vi "Normalize 1D float array.vi"(10 "Signal treat":T1(ring), 11 "Data in":sgl[](array[numeric])) -> (3 "Data out":sgl[](array[numeric]))   [LabVIEW 2021, in "MatS Libs.lvlib"]
doc: "Scales signal in 1D array of single precision numbers.\nFor double precision, you can use Scale.vi, Quick scale.vi or Normalize.vi from Signal processing palete."
uses:
  <userlib>/_MGI/1D Array/MGI Average/MGI Average (SGL[]).vi
  <userlib>/MatS Libs/MatS Libs.lvlib
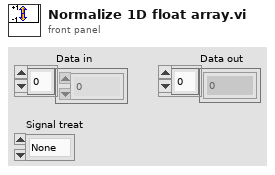
[diagram p1: front panel]
types:
  T1 = enum16{"None", "Unity norm", "Mean norm", "Standardization"}
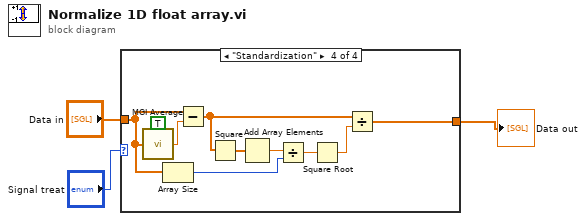
[diagram p0: block diagram]
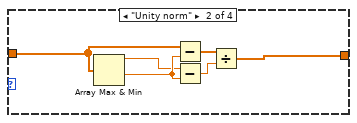
[diagram p3: hidden frame]
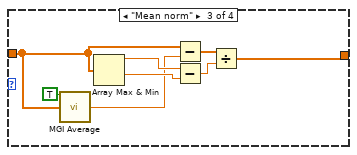
[diagram p4: hidden frame]
diagram:
  n1 = case shown="\"Standardization\"" "Signal treat" {
    tunnel: [w4 w8 w13 w26] -> w3
    tunnel: "Data in" -> [w4 w10 w16 w23]
    frame "None", Default {
      # "No feature scaling"
    }
    frame "Unity norm" {
      n2 = Array Max & Min(array=w10) -> (max value=w7:sgl, min value=w9:sgl)  [unwired: 2 out]
      n3 = Subtract(x=w10, y=w9) -> (x-y=w6:sgl[])
      n4 = Subtract(x=w7, y=w9) -> (x-y=w5:sgl)
      n5 = Divide(x=w6, y=w5) -> (x/y=w8:sgl[])
    }
    frame "Mean norm" {
      n6 = call-poly <userlib>:"MGI Average.vi"("Single[]"=w16, "Ignore NaN? (F)"=TRUE) -> ("Average"=w15:sgl)
      n7 = Array Max & Min(array=w16) -> (max value=w17:sgl, min value=w18:sgl)  [unwired: 2 out]
      n8 = Subtract(x=w16, y=w15) -> (x-y=w12:sgl[])
      n9 = Subtract(x=w17, y=w18) -> (x-y=w11:sgl)
      n10 = Divide(x=w12, y=w11) -> (x/y=w13:sgl[])
    }
    frame "Standardization" {
      n11 = call-poly <userlib>:"MGI Average.vi"("Single[]"=w23, "Ignore NaN? (F)"=TRUE) -> ("Average"=w28:sgl)
      n12 = Array Size(array=w23) -> (size(s)=w20:i32)
      n13 = Subtract(x=w23, y=w28) -> (x-y=w24:sgl[])
      n14 = Square(x=w24) -> (x^2=w21:sgl[])
      n15 = Add Array Elements(numeric array=w21) -> (sum=w22:sgl)
      n16 = Divide(x=w22, y=w20) -> (x/y=w19:sgl)
      n17 = Square Root(x=w19) -> (sqrt(x)=w25:sgl)
      n18 = Divide(x=w24, y=w25) -> (x/y=w26:sgl[])
    }
  }
  "Data out" <- w3
